vi "Robot Global Data.vi"() -> ()   [LabVIEW 2015]
doc: "This global VI can contain as many global variables as you need. Place a control on the panel, give it a good name. To read or write to it from a VI, drag the icon to the diagram of that VI. You can also drag from the project. Click on the node to change which global you access. You shouldn't have multiple locations writing to a global or it will cause a race-condition."
uses:
  <vilib>/Rock Robotics/WPI/Camera/WPI_CameraImageSize.ctl
  <vilib>/Rock Robotics/WPI/DriverStation/WPI_DriverStationRobotMode2.ctl
panel:
  in  "Hall Effect Count Value":i32
  in  "Arm Movement Parameters":T1
  in  "Arm Async Enabled":bool
  in  "Arm Task Mode":enum16{"Synchronous", "Asynchronous"}(ring)
  in  "Arm Direction":enum16{"Up", "Down"}(ring)
  in  "Drive Async Parameters":T2
  in  "Gyro Rate":dbl(graph)
  in  "Drive Task Mode":enum16{"Synchronous", "Asynchronous"}(ring)
  in  "Gyro Angle":dbl
  in  "Drive Async Enabled":bool
  in  "Simulated":bool
  in  "Robot Mode":T3
  in  "image size":T4=enum."320x240"
  in  "Enable Vision":bool
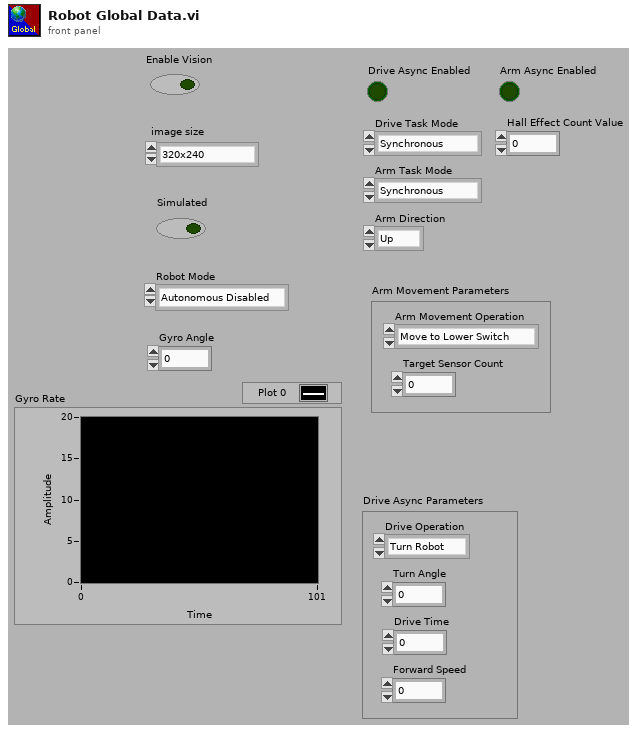
[diagram p1: front panel]
types:
  T1 = cluster{"Arm Movement Operation":enum16{"Move to Lower Switch", "Move to Upper Switch", "Move to Sensor Count"}, "Target Sensor Count":i32}
  T2 = cluster{"Drive Operation":enum16{"Turn Robot", "Drive Straight for Time"}, "Turn Angle":dbl, "Drive Time":dbl, "Forward Speed":dbl}
  T3 = typedef "WPI_DriverStationRobotMode2.ctl" = enum16{"Autonomous Disabled", "Autonomous Enabled", "Teleop Disabled", "Teleop Enabled", "Disconnected", "Finish", "Test Disabled", "Test Enabled", "Emergency Stopped"}
  T4 = typedef "WPI_CameraImageSize.ctl" = enum16{"640x480", "320x240", "160x120", "Custom"}
diagram:
